vi "4145 Receive Message.vi"(5 "source":string, 6 "timeout ms":u32=25000, 7 "error in":T2, 8 "read mode":i32(ring) items=["terminate read on EOI or byte count", "terminate read on EOI, byte count, or CR", "terminate read on EOI, byte count, or LF"], 9 "byte count in":i32, 10 "4145_GPIB_COM_ctrl":T1={"Address_string"="17", "timeout ms"=25000, "Terminator"=",", "LoggerQueue"=refnum}) -> (0 "error out":T2, 1 "status OUT":bool[](array[boolean]), 2 "read buffer OUT":string, 3 "4145_GPIB_COM_ctrl 2":T1={"Address_string"="17", "timeout ms"=25000, "Terminator"=",", "LoggerQueue"=refnum})   [LabVIEW 2014]
doc: "Sends a string to a message based VXI instrument. In order to communicate with an instrument, you must first open the instrument by running the Open VXI Instrument or running the initialize VI (initialize VIs call the Open VXI Instrument in their block diagram). Use the instrument ID generated by the Open VXI Instrument to address the specific instrument, then set the write mode and enter the string to send. If a write error occurs, error code 1230 is returned. If you fail to open the instrument, error code 1232 is returned."
uses:
  typedef/4145_GPIB_Com.ctl
  typedef/4145_que_msg.ctl
  typedef/4145 command enum.ctl
panel:
  in  "status IN":bool[](array[boolean])
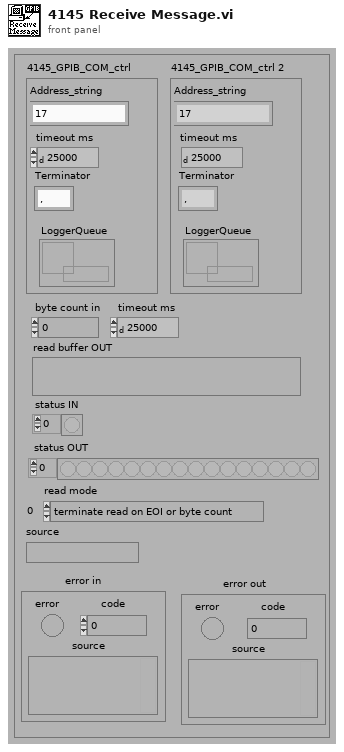
[diagram p1: front panel]
types:
  T1 = typedef "4145_GPIB_Com.ctl" = cluster{"Address_string":string, "timeout ms":u32, "Terminator":string, "LoggerQueue":refnum<queue>}
  T2 = cluster{"error":bool, "code":i32, "source":string}
  T3 = typedef "4145 command enum.ctl" = enum16{"DEFAULT", "INFORMATION", "ERROR", "STATUS", "CAUTION", "WARNING", "OFFLINE", "STOP"}
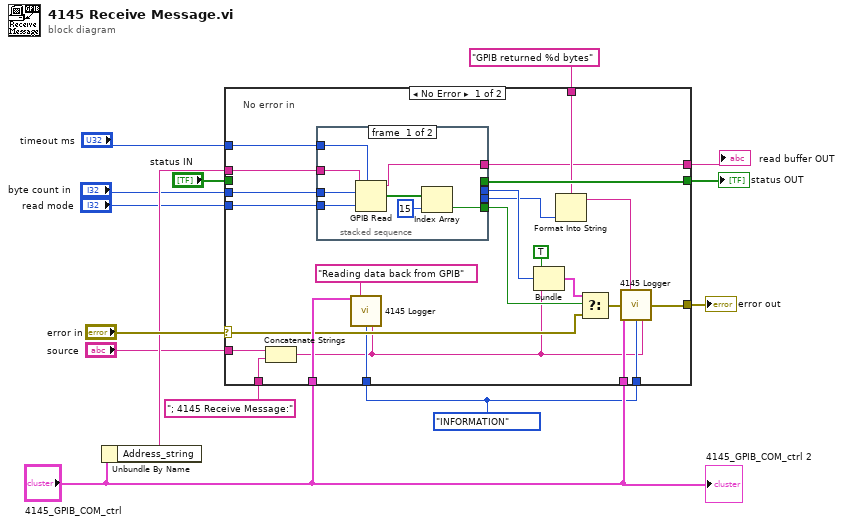
[diagram p0: block diagram]
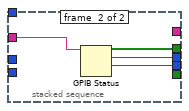
[diagram p2: hidden frame]
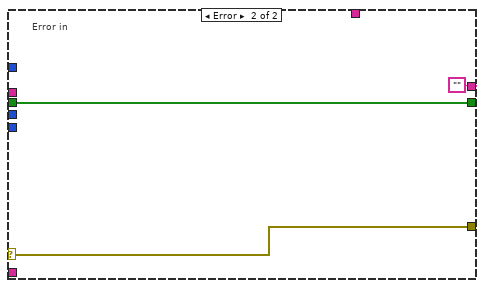
[diagram p3: hidden frame]
diagram:
  w2 = 4145_command_enum."INFORMATION" ("msg_type")
  n1 = Unbundle By Name("4145_GPIB_COM_ctrl") -> ("Address_string"=w10:string)
  n2 = case shown="No Error" "error in" {
    selector: "error in" -> [w27 w52]
    tunnel: "status IN" -> [_ w53]
    tunnel: [w36 w53] -> w14
    tunnel: [w22 w52] -> w12
    tunnel: w10 -> [w35 _]
    tunnel: "; 4145 Receive Message:" -> [w34 _]
    tunnel: "source" -> [w33 _]
    tunnel: "timeout ms" -> [w32 _]
    tunnel: "byte count in" -> [w31 _]
    tunnel: "read mode" -> [w30 _]
    tunnel: "4145_GPIB_COM_ctrl" -> [w29 _]
    tunnel: "4145_GPIB_COM_ctrl" -> [w28 _]
    tunnel: w2 -> [w26 _]
    tunnel: "GPIB returned %d bytes" -> [w20 _]
    tunnel: w2 -> [w18 _]
    tunnel: [w16 ""] -> w1
    frame No Error {
      # "No error in"
      n3 = Concatenate Strings(w33, w34) -> (w17:string)
      n4 = stacked-sequence {
        tunnel: [_ w50] -> w36
        tunnel: [w44 _] -> w37
        tunnel: [_ w49] -> w21
        tunnel: w35 -> [w43 w48]
        tunnel: w32 -> [w42 _]
        tunnel: w30 -> [w41 _]
        tunnel: w31 -> [w40 _]
        tunnel: [w39 _] -> w16
        tunnel: [_ w47] -> w15
        frame #0 {
          n5 = GPIB Read(0:w43, 1:w40, 2:w41, 4:w42) -> (5:w39:string, 6:w45:bool[])  [unwired: 1 in, 1 out]
          n6 = Index Array(array=w45, index=15) -> (element=w44:bool)
        }
        frame #1 {
          n7 = GPIB Status(0:w48) -> (2:w50:bool[], 3:w49:i16, 4:w47:i32)  [unwired: 1 in, 1 out]
        }
      }
      n8 = call "4145 Logger.vi"("4145_GPIB_COM_ctrl"=w28, "msg"="Reading data back from GPIB", "msg_type"=w26, "origin vi"=w17) -> ()  [unwired: 11 in, 1 out]
      n9 = Bundle(TRUE, "GPIB error"=w21, w17) -> (w24:cluster{bool, "GPIB error":i16, string})  [unwired: 1 in]
      n10 = Format Into String(format string=w20, w15) -> (resulting string=w19:string)  [unwired: 2 in, 1 out]
      n11 = Select(t=w24, s=w37, f=w27) -> (s? t:f=w23:errorcluster)
      n12 = call "4145 Logger.vi"("4145_GPIB_COM_ctrl"=w29, "msg"=w19, "msg_type"=w18, "origin vi"=w17, "error in (no error)"=w23) -> ("error out"=w22:errorcluster)  [unwired: 10 in]
    }
    frame Error {
      # "Error in"
    }
  }
  "status OUT" <- w14
  "error out" <- w12
  "read buffer OUT" <- w1
  "4145_GPIB_COM_ctrl 2" <- "4145_GPIB_COM_ctrl"
